vi "updateStateList.vi"(8 "error in (no error)":errorcluster, 11 "StaticOutputEditor in":refnum<class "StaticOutputEditor.lvclass">) -> (0 "error out":errorcluster, 3 "StaticOutputEditor out":refnum<class "StaticOutputEditor.lvclass">)   [LabVIEW 2009, in "Views.lvlib" / "ScriptEditor.lvlib" / "StaticOutputEditor.lvclass"]
uses:
  StaticOutputEditor.lvclass
  StaticOutputEditor.lvclass/StaticOutputEditor.ctl
  Tools/DatabaseHelpers/Database Objects/ChannelArray/ChannelArray.lvclass
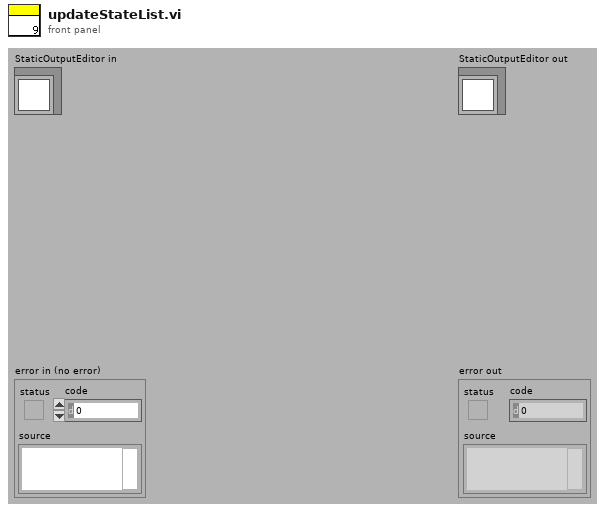
[diagram p1: front panel]
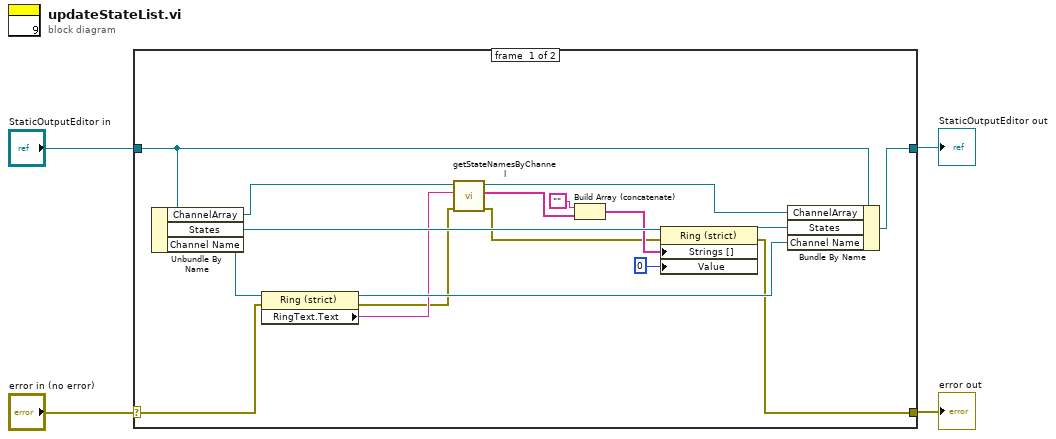
[diagram p0: block diagram]
diagram:
  n1 = case shown="No Error" "error in (no error)" {
    selector: "error in (no error)" -> [w19 w23]
    tunnel: [w13 w23] -> w3
    tunnel: [w5 w22] -> w1
    tunnel: "StaticOutputEditor in" -> [w7 w22]
    frame #0 {
      n2 = Unbundle By Name(w7) -> ("ChannelArray"=w12:refnum<class "ChannelArray.lvclass">, "States"=w18:refnum<vi>, "Channel Name"=w21:refnum<vi>)
      n3 = property class="Ring (strict)"(reference=w21, error in=w19) -> (reference out=w20:refnum<vi>, error out=w9:errorcluster, "RingText.Text"=w10:string)
      n4 = call "getStateNamesByChannel.vi"("error in (no error)"=w9, "channel_name"=w10, "ChannelArray in"=w12) -> ("error out"=w8:errorcluster, "state_names"=w11:string[], "ChannelArray out"=w6:refnum<class "ChannelArray.lvclass">)  [unwired: 6 in]
      n5 = Build Array (concatenate)("", w11) -> (w16:string[])
      n6 = property class="Ring (strict)"(reference=w18, error in=w8, "Strings []"=w16, "Value"=0) -> (reference out=w14:refnum<vi>, error out=w13:errorcluster)
      n7 = Bundle By Name(cluster=w7, "ChannelArray"=w6, "States"=w14, "Channel Name"=w20) -> (w5:refnum<class "StaticOutputEditor.lvclass">)
    }
    frame #1 {
    }
  }
  "error out" <- w3
  "StaticOutputEditor out" <- w1
